vi "Open Serial Port.vi"(8 "error in (no error)":errorcluster, 9 "Serial Configuraiton":T1={"timeout ms"=10000, "data bits"=8, "parity"=enum."None", "baud rate"=9600, "stop bits"=10, "flow control"=0} {"stop bits" items=["1.0"=10, "1.5"=15, "2.0"=20]; "flow control" items=["None", "XON/XOFF", "RTS/CTS", "XON/XOFF & RTS/CTS", "DTR/DSR", "XON/XOFF & DTR/DSR"]}, 10 "VISA resource":refnum<visa-resource-name>, 11 "Gantry in":refnum<class "Gantry.lvclass">) -> (0 "error out":errorcluster, 2 "Connection ID":i32, 3 "Gantry out":refnum<class "Gantry.lvclass">)   [LabVIEW 2023, in "Gantry.lvclass"]
uses:
  Gantry.lvclass
  Gantry.lvclass/Gantry.ctl
  <vilib>/Instr/_visa.llb/VISA Configure Serial Port (Serial Instr).vi
  Type Definitions/Serial Configuration.ctl
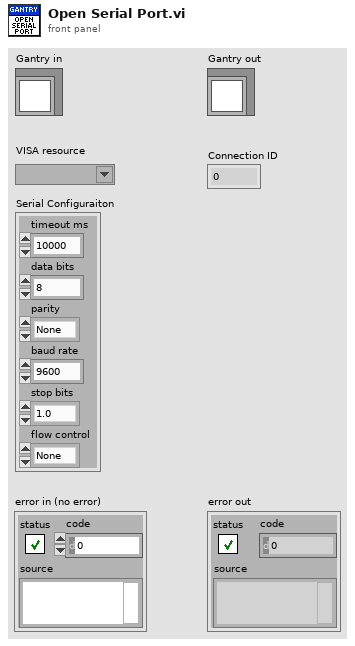
[diagram p1: front panel]
types:
  T1 = typedef "Serial Configuration.ctl" = cluster{"timeout ms":u32, "data bits":u16, "parity":enum16{"None", "Odd", "Even", "Mark", "Space"}, "baud rate":u32, "stop bits":u16, "flow control":u16}
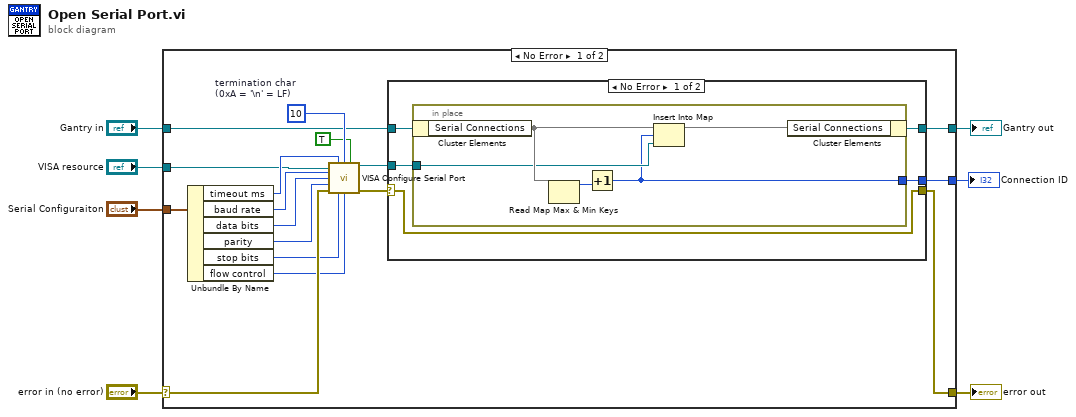
[diagram p0: block diagram]
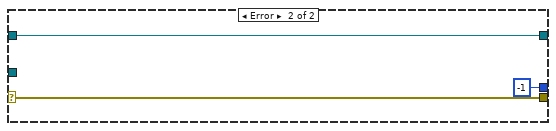
[diagram p2: hidden frame]
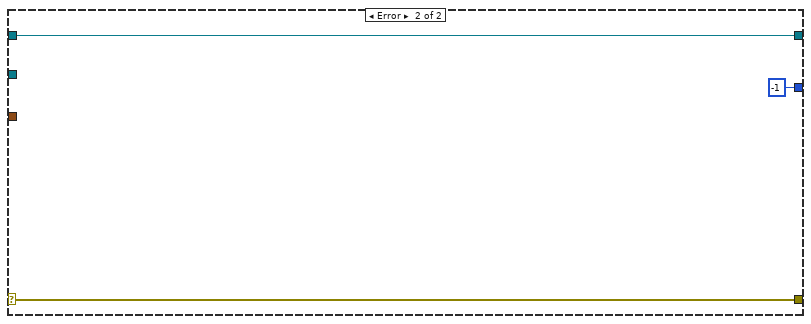
[diagram p3: hidden frame]
diagram:
  n1 = case shown="No Error" "error in (no error)" {
    selector: "error in (no error)" -> [w24 w40]
    tunnel: [w12 w40] -> w6
    tunnel: [w11 w39] -> w4
    tunnel: "Gantry in" -> [w14 w39]
    tunnel: "Serial Configuraiton" -> [w22 _]
    tunnel: [w9 -1] -> w2
    tunnel: "VISA resource" -> [w8 _]
    frame No Error {
      w23 = u8 10  # termination char (0xA = '\n' = LF)
      n2 = Unbundle By Name(w22) -> ("timeout ms"=w21:u32, "baud rate"=w20:u32, "data bits"=w19:u16, "parity"=w18:enum16{"None", "Odd", "Even", "Mark", "Space"}, "stop bits"=w17:u16, "flow control"=w16:u16)
      n3 = call-poly "VISA Configure Serial Port"("VISA resource name"=w8, "timeout (10sec)"=w21, "termination char\n(0xA = '\\n' = LF)"=w23, "Enable Termination\nChar (T)"=TRUE ("Enable Termination\nChar (T)"), "baud rate (9600)"=w20, "data bits (8)"=w19, "parity (0:none)"=w18, "error in (no error)"=w24, "stop bits (10: 1 bit)"=w17, "flow control (0:none)"=w16) -> ("VISA resource name out"=w10:refnum<visa-resource-name>, "error out"=w13:errorcluster)  [unwired: 4 in]
      n4 = case shown="No Error" w13 {
        selector: w13 -> [w26 w37]
        tunnel: w14 -> [w29 w36]
        tunnel: [w26 w37] -> w12
        tunnel: [w25 w36] -> w11
        tunnel: w10 -> [w28 _]
        tunnel: [w27 -1] -> w9
        frame No Error {
          n5 = in-place {
            in-place-border: w28 -> [w32]
            in-place-border: [w30] -> w27
            n6 = in-place-cluster #1(w29) -> ("Serial Connections"=w33:map{i32, refnum<visa-resource-name>})
            n7 = Read Map Max & Min Keys(11:w33) -> (3:w34:i32)  [unwired: 1 out]
            n8 = Increment(x=w34) -> (x+1=w30:i32)
            n9 = Insert Into Map(map in=w33, key=w30, value=w32) -> (map out=w31:map{i32, refnum<visa-resource-name>})  [unwired: 2 out]
            n10 = in-place-cluster #1("Serial Connections"=w31) -> (w25:refnum<class "Gantry.lvclass">)
          }
        }
        frame Error {
        }
      }
    }
    frame Error {
    }
  }
  "error out" <- w6
  "Gantry out" <- w4
  "Connection ID" <- w2
